vi "Test Class YOLO.vi"() -> ()   [LabVIEW 2017]
doc: "Created IvanLis by LabVIEW Portal\nProfile: http://labviewportal.org/memberlist.php?mode=viewprofile&u=987\neMail: IvanLisanov@gMail.com\nTelegram: https://t.me/IvanLis"
uses:
  ONNX YOLO Class/ONNX YOLO Class.lvclass
  ONNX YOLO Class/TypeDef/Circle.ctl
  ONNX YOLO Class/ONNX YOLO Class Library.lvlib
  ONNX Class/TypeDef/IO.ctl
  ONNX Class/ONNX Class Library.lvlib
  ONNX Class/TypeDef/Introspection.ctl
panel:
  out "Circles":T1[](array[typedef])
  out "count":i32
  out "2D Picture":picture
  in  "Auto Clear Buffer":bool
  in  "Auto Init Buffer":bool=TRUE
  out "Metadata":string[][](table)
  out "Introspection Output":T2
  out "Introspection Input":T2
  out "error out":errorcluster
  in  "Auto UnLoad":bool
  out "ONNX Path":path
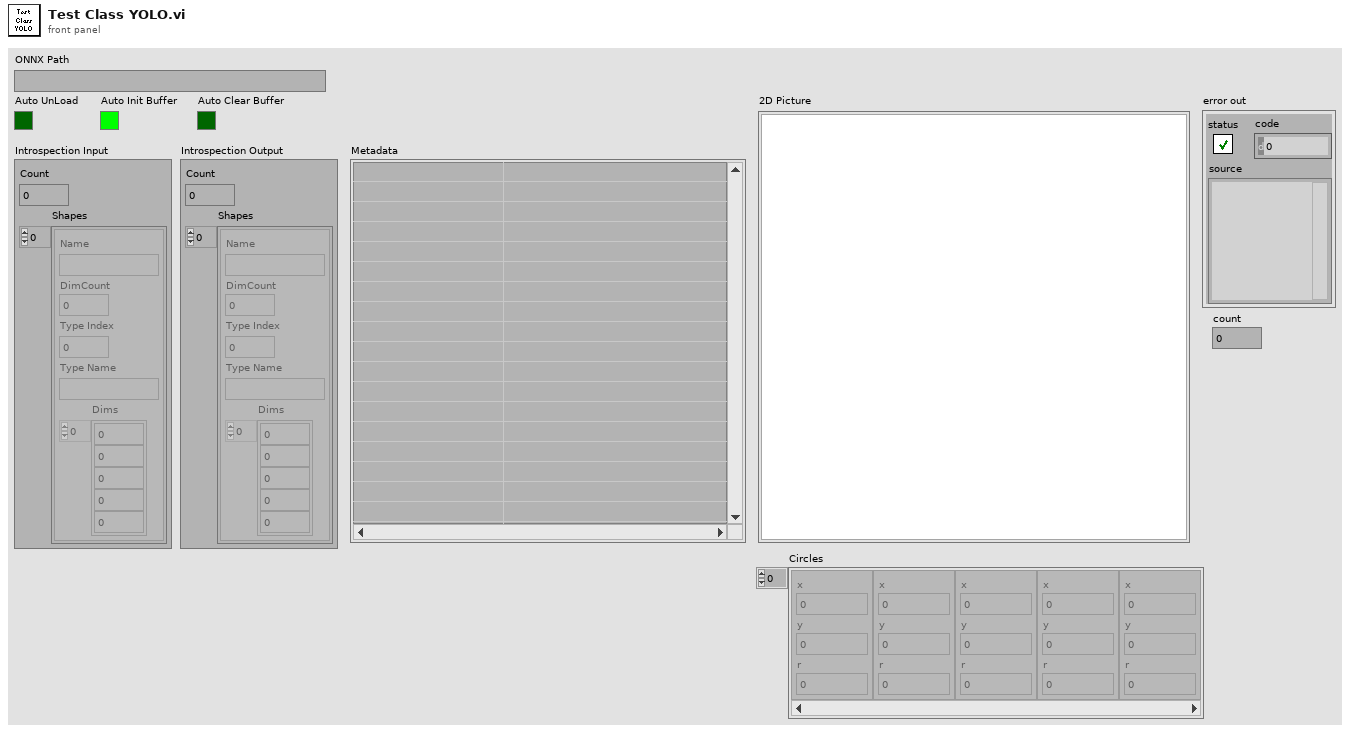
[diagram p1: front panel]
types:
  T1 = typedef "ONNX YOLO Class Library.lvlib/Circle.ctl" = cluster{"x":sgl, "y":sgl, "r":sgl}
  T2 = typedef "ONNX Class Library.lvlib/Introspection.ctl" = cluster{"Count":i32, "Shapes":T3[]}
  T3 = typedef "ONNX Class Library.lvlib/IO.ctl" = cluster{"Name":string, "DimCount":i32, "Type Index":i32, "Type Name":string, "Dims":i64[]}
  T4 = typedef "imagedata.ctl" = cluster{"image type":i32, "image depth":i32, "image":u8[], "mask":u8[], "colors":u32[], "Rectangle":cluster{"left":i16, "top":i16, "right":i16, "bottom":i16}}
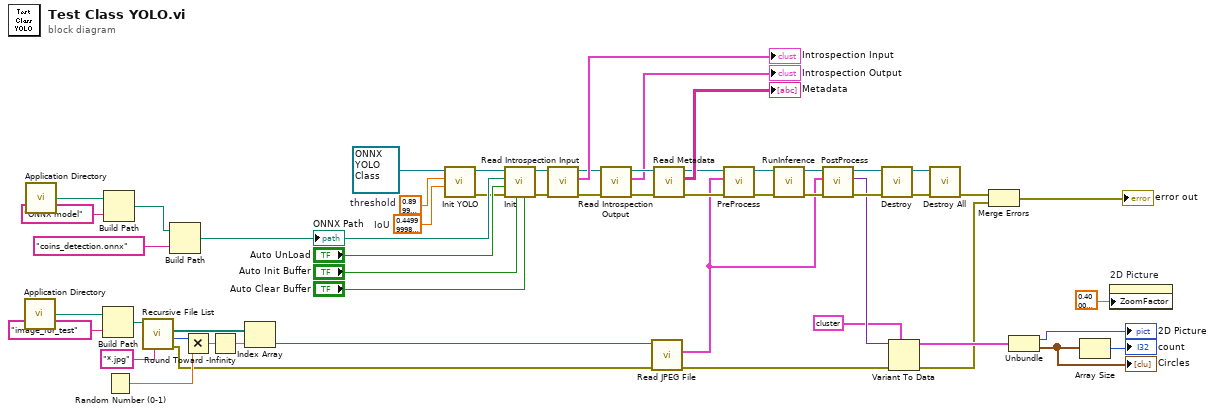
[diagram p0: block diagram]
diagram:
  w35 = sgl 0.45  # IoU
  w36 = sgl 0.9  # threshold
  n1 = call <vilib>:"Application Directory.vi"() -> ("Application Directory"=w10:path)
  n2 = call <vilib>:"Application Directory.vi"() -> ("Application Directory"=w51:path)
  n3 = Build Path(base path=w10, name or relative path="image_for_test") -> (appended path=w9:path)
  n4 = Build Path(base path=w51, name or relative path="ONNX model") -> (appended path=w49:path)
  n5 = Random Number (0-1)() -> (number: 0 to 1=w7:dbl)
  n6 = call <vilib>:"Recursive File List.vi"("pattern"="*.jpg", "Folder Path"=w9) -> ("error out"=w2:errorcluster, "Number of Files"=w6:i32, "All Files in Dir"=w4:path[])  [unwired: 5 in, 2 out]
  n7 = Build Path(base path=w49, name or relative path="coins_detection.onnx") -> (appended path=w48:path)
  "ONNX Path" <- w48
  n8 = Multiply(x=w6, y=w7) -> (x*y=w5:dbl)
  n9 = Round Toward -Infinity(1:w5) -> (0:w3:dbl)
  n10 = Index Array(array=w4, index=w3) -> (element=w1:path)
  n11 = call-dynamic "Init YOLO.vi"("IoU"=w35, "threshold"=w36, "ONNX YOLO Class in"=refnum<class "ONNX YOLO Class.lvclass"> refnum) -> ("error out"=w37:errorcluster, "ONNX YOLO Class out"=w38:refnum<class "ONNX YOLO Class.lvclass">)  [unwired: 7 in]
  n12 = call-dynamic "Init.vi"("Auto Clear Buffer"="Auto Clear Buffer", "Auto Init Buffer"="Auto Init Buffer", "error in (no error)"=w37, "Auto UnLoad"="Auto UnLoad", "ONNX Path"=w48, "ONNX Class in"=w38) -> ("error out"=w45:errorcluster, "ONNX Class out"=w46:refnum<class "ONNX YOLO Class.lvclass">)  [unwired: 3 in, 1 out]
  n13 = call-dynamic "Read Introspection Input.vi"("error in (no error)"=w45, "ONNX Class in"=w46) -> ("error out"=w25:errorcluster, "Introspection"=→"Introspection Input":T2, "ONNX Class out"=w27:refnum<class "ONNX YOLO Class.lvclass">)  [unwired: 7 in]
  n14 = call-dynamic "Read Introspection Output.vi"("error in (no error)"=w25, "ONNX Class in"=w27) -> ("error out"=w28:errorcluster, "Introspection"=→"Introspection Output":T2, "ONNX Class out"=w26:refnum<class "ONNX YOLO Class.lvclass">)  [unwired: 7 in]
  n15 = call <vilib>:"Read JPEG File.vi"("error in (no error)"=w2, "path to JPEG file"=w1) -> ("error out"=w19:errorcluster, "image data"=w20:T4)  [unwired: 7 in, 1 out]
  n16 = call-dynamic "Read Metadata.vi"("error in (no error)"=w28, "ONNX Class in"=w26) -> ("error out"=w33:errorcluster, "Metadata"=→"Metadata":string[][], "ONNX Class out"=w34:refnum<class "ONNX YOLO Class.lvclass">)  [unwired: 7 in]
  n17 = call-dynamic "PreProcess.vi"("error in (no error)"=w33, "Variant in"=w20, "ONNX YOLO Class in"=w34) -> ("error out"=w22:errorcluster, "ONNX YOLO Class out"=w23:refnum<class "ONNX YOLO Class.lvclass">)  [unwired: 6 in, 1 out]
  n18 = call-dynamic "RunInference.vi"("error in (no error)"=w22, "ONNX Class in"=w23) -> ("error out"=w31:errorcluster, "ONNX Class out"=w32:refnum<class "ONNX YOLO Class.lvclass">)  [unwired: 7 in, 1 out]
  n19 = call-dynamic "PostProcess.vi"("error in (no error)"=w31, "Variant in"=w20, "ONNX YOLO Class in"=w32) -> ("error out"=w29:errorcluster, "Variant out"=w18:variant, "ONNX YOLO Class out"=w30:refnum<class "ONNX YOLO Class.lvclass">)  [unwired: 6 in]
  n20 = call-dynamic "Destroy.vi"("error in (no error)"=w29, "ONNX Class in"=w30) -> ("error out"=w54:errorcluster, "ONNX Class out"=w55:refnum<class "ONNX YOLO Class.lvclass">)  [unwired: 8 in]
  n21 = Variant To Data(error in=w19, type=cluster{"new picture":picture, T1[]} {"new picture"=bytes[0], []} ("output cluster"), Variant=w18) -> (data=w16:cluster{"new picture":picture, T1[]}, error out=w12:errorcluster)
  n22 = call-dynamic "Destroy All.vi"("error in (no error)"=w54, "ONNX Class in"=w55) -> ("error out"=w47:errorcluster)  [unwired: 8 in, 1 out]
  n23 = Merge Errors(w47, w12) -> (→"error out":errorcluster)
  n24 = Unbundle(w16) -> ("new picture"=→"2D Picture":picture, w14:T1[])
  "Circles" <- w14
  n25 = Array Size(array=w14) -> (size(s)=→"count":i32)
  n26 = property on="2D Picture" class="Pict"("ZoomFactor"=sgl 0.4 ("Zoom Factor")) -> ()  [unwired: 2 in, 2 out]
